vi "Update Busy LED.vi"(6 "Assert After (500 ms)":u32=500, 7 "RUNNING Ref":refnum<vi>, 8 "error in (no error)":errorcluster, 10 "Busy (False)":bool, 11 "BUSY Ref":refnum<vi>) -> (0 "error out":errorcluster)   [LabVIEW 2025, in "I2C Bus Monitor UI.lvlib"]
uses:
  I2C Bus Monitor UI.lvlib
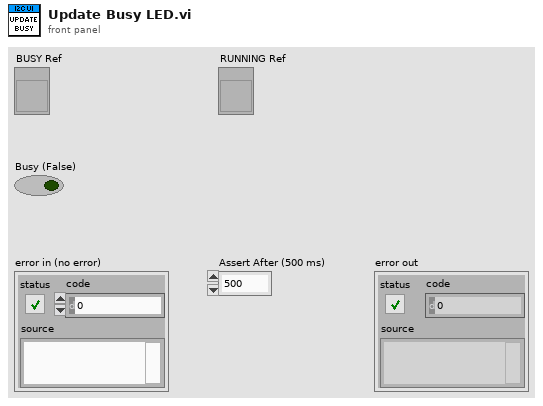
[diagram p1: front panel]
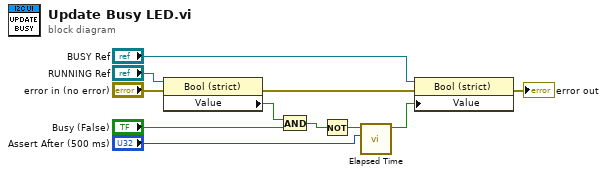
[diagram p0: block diagram]
diagram:
  n1 = property class="Bool (strict)"(reference="RUNNING Ref", error in="error in (no error)") -> (error out=w4:errorcluster, "Value"=w2:bool)  [unwired: 1 out]
  n2 = And(x=w2, y="Busy (False)") -> (x .and. y?=w3:bool)
  n3 = Not(x=w3) -> (.not. x?=w5:bool)
  n4 = call "Elapsed Time.vi"("Target (ms)"="Assert After (500 ms)", "Reset"=w5) -> ("Elapsed"=w9:bool)  [unwired: 8 in, 1 out]
  n5 = property class="Bool (strict)"(reference="BUSY Ref", error in=w4, "Value"=w9) -> (error out=→"error out":errorcluster)  [unwired: 1 out]
